vi "clear_software_buffer.vi"(8 "error in (no error)":errorcluster, 11 "GenericDAQ in":refnum<class "GenericDAQ.lvclass">) -> (0 "error out":errorcluster, 3 "GenericDAQ out":refnum<class "GenericDAQ.lvclass">)   [LabVIEW 2017, in "GenericDAQ.lvclass"]
uses:
  GenericDAQ.lvclass
  GenericDAQ.lvclass/GenericDAQ.ctl
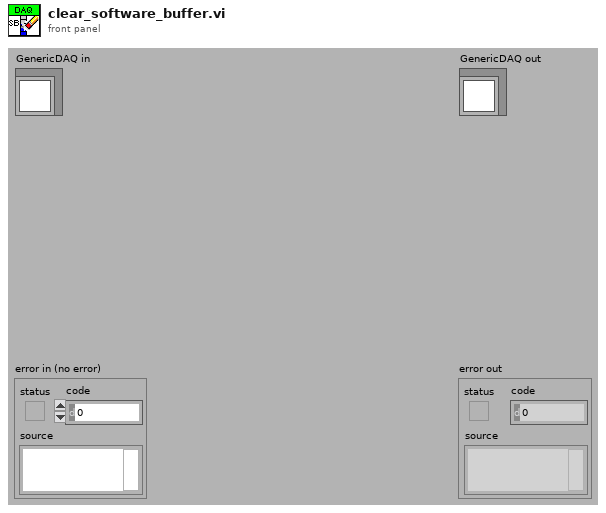
[diagram p1: front panel]
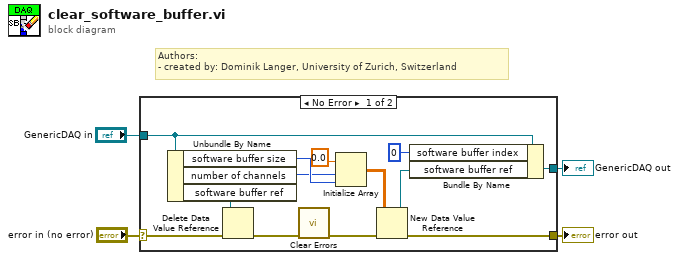
[diagram p0: block diagram]
diagram:
  # "Authors: \n- created by: Dominik Langer, University of Zurich, Switzerland"
  n1 = case shown="No Error" "error in (no error)" {
    selector: "error in (no error)" -> [w8 w19]
    tunnel: [w12 w19] -> w3
    tunnel: [w11 w18] -> w2
    tunnel: "GenericDAQ in" -> [w7 w18]
    frame No Error {
      n2 = Unbundle By Name(w7) -> ("software buffer size"=w15:i32, "number of channels"=w14:i32, "software buffer ref"=w9:refnum<data-value>)
      n3 = Delete Data Value Reference(data value reference=w9, error in=w8) -> (error out=w6:errorcluster)  [unwired: 1 out]
      n4 = call <vilib>:"Clear Errors.vi"("error in (no error)"=w6) -> ("error out"=w5:errorcluster)  [unwired: 5 in, 1 out]
      n5 = Initialize Array(0.0, w14, w15) -> (w17:dbl[][])
      n6 = New Data Value Reference(data value=w17, error in=w5) -> (data value reference=w13:refnum<data-value>, error out=w12:errorcluster)
      n7 = Bundle By Name(cluster=w7, "software buffer index"=0, "software buffer ref"=w13) -> (w11:refnum<class "GenericDAQ.lvclass">)
    }
    frame Error {
    }
  }
  "error out" <- w3
  "GenericDAQ out" <- w2
